vi "Instantiate dotNET Container.vi"(8 "error in (no error)":errorcluster, 11 "Panel Reference":refnum<k24>(container)) -> (0 "error out":errorcluster, 3 "dotNET Container out":refnum<class "dotNET Container.lvclass">)   [LabVIEW 2019, in "dotNET Container.lvclass"]
uses:
  dotNET Container.lvclass
  D:/Namratha/MDI/LabVIEW-MDI-develop_LV2019/source code/Container/Container base/Container base.lvclass
  Container base/Container base.lvclass/Container base.ctl
  Container base/property/Write HWND.vi
  System.Windows.Forms
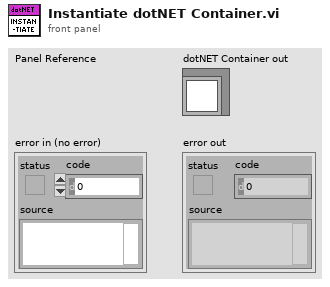
[diagram p1: front panel]
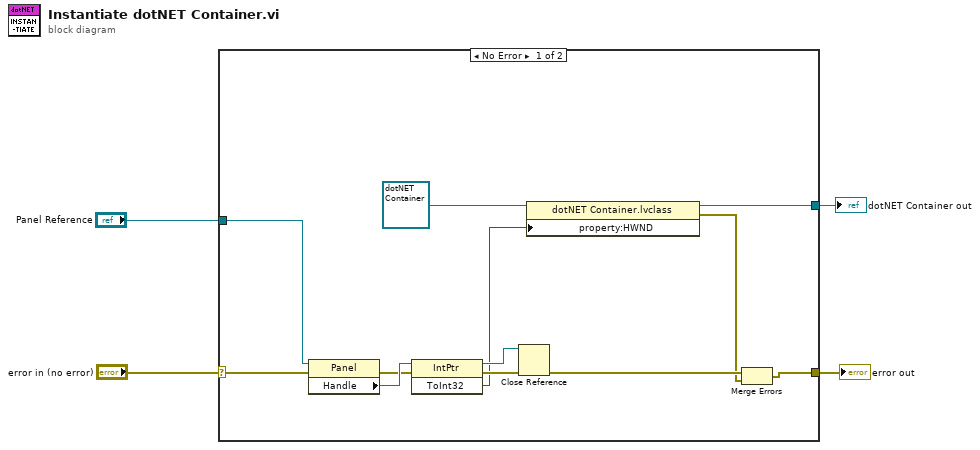
[diagram p0: block diagram]
diagram:
  n1 = case shown="No Error" "error in (no error)" {
    selector: "error in (no error)" -> [w11 w17]
    tunnel: [w6 w17] -> w3
    tunnel: "Panel Reference" -> [w12 _]
    tunnel: [w7 _] -> w1
    frame No Error {
      n2 = property class="Panel"(reference=w12, error in=w11) -> (error out=w15:errorcluster, "Handle"=w16:refnum<k24>)  [unwired: 1 out]
      n3 = invoke class="IntPtr" method="ToInt32"(reference=w16, error in=w15) -> (reference out=w13:refnum<k24>, error out=w14:errorcluster, "ToInt32"=w8:i32)  [unwired: 1 in]
      n4 = Close Reference(reference=w13, error in (no error)=w14) -> (error out=w10:errorcluster)
      n5 = property class="dotNET Container.lvclass"(reference=refnum<class "dotNET Container.lvclass"> refnum ("dotNET Container out"), "property:HWND"=w8) -> (reference out=w7:refnum<class "dotNET Container.lvclass">, error out=w5:errorcluster)  [unwired: 1 in]
      n6 = Merge Errors(w10, w5) -> (w6:errorcluster)
    }
    frame Error {
    }
  }
  "error out" <- w3
  "dotNET Container out" <- w1
